vi "Get RegistrationRequest.vi"(8 "error in (no error)":errorcluster, 11 "gRPCid in":T1) -> (0 "error out":errorcluster, 2 "Request Data":T2, 3 "gRPCid out":T1)   [LabVIEW 2019]
uses:
  RegistrationRequest_Data.ctl
  gRPC interface/Server API/typeDefs/grpcId.ctl
  905457ba-43ee-4d7e-b70e-0cf7ac2d3d08.vi
  gRPC interface/gprc-lvsupport.lvlib
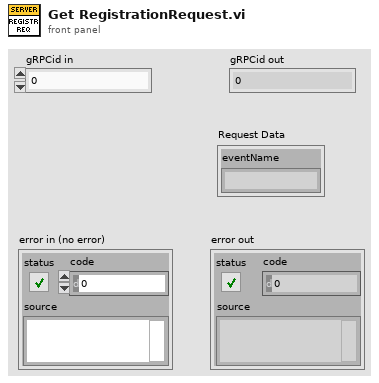
[diagram p1: front panel]
types:
  T1 = typedef "gprc-lvsupport.lvlib/grpcId.ctl" = u64
  T2 = typedef "RegistrationRequest_Data.ctl" = cluster{"eventName":string}
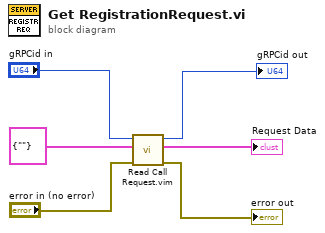
[diagram p0: block diagram]
diagram:
  n1 = call "Read Call Request.vim"("error in (no error)"="error in (no error)", "Data Type"=T2 {"eventName"=""} ("RegistrationRequest_Data"), "gRPCid in"="gRPCid in") -> ("error out"=→"error out":errorcluster, "Request Data"=→"Request Data":T2, "gRPCid out"=→"gRPCid out":T1)  [unwired: 6 in]
